vi "CoilsInit.vi"(8 "error in":errorcluster, 9 "DO Lines":tag, 10 "AO Channels":tag, 11 "Keithley USB":refnum<visa-resource-name>) -> (0 "error out":errorcluster, 1 "DO Task out":refnum<k21>, 2 "AO Task out":refnum<k21>, 3 "Keithley USB out":refnum<visa-resource-name>)   [LabVIEW 2012]
uses:
  <vilib>/DAQmx/create/channels.llb/DAQmx Create Channel (AO-Voltage-Basic).vi
  <vilib>/DAQmx/create/channels.llb/DAQmx Create Channel (DO-Digital Output).vi
  <resource>/objmgr/daqmx.rc
  Keithley KE22xx Series/Keithley KE22xx Series.lvlib
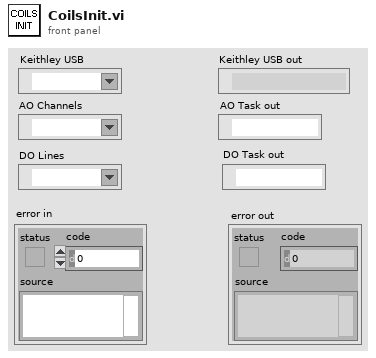
[diagram p1: front panel]
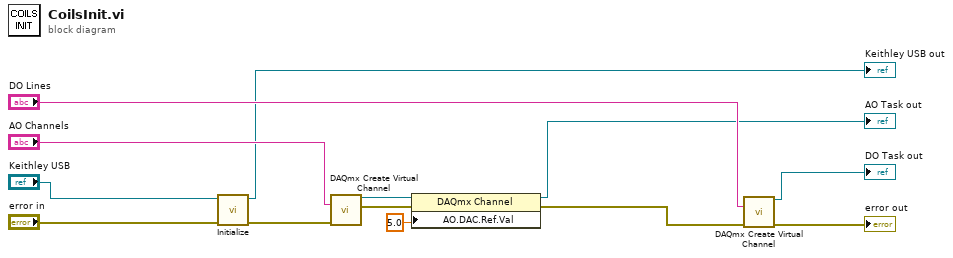
[diagram p0: block diagram]
diagram:
  n1 = call "Initialize.vi"("error in (no error)"="error in", "VISA resource name"="Keithley USB") -> ("error out"=w9:errorcluster, "VISA resource name out"=→"Keithley USB out":refnum<visa-resource-name>)  [unwired: 8 in]
  n2 = call-poly <vilib>:"DAQmx Create Virtual Channel.vi"("physical channels"="AO Channels", "error in"=w9) -> ("task out"=w12:refnum<k21>, "error out"=w11:errorcluster)  [unwired: 12 in]
  n3 = property class="DAQmx Channel"(reference=w12, error in=w11, "AO.DAC.Ref.Val"=5.0) -> (reference out=→"AO Task out":refnum<k21>, error out=w8:errorcluster)
  n4 = call-poly <vilib>:"DAQmx Create Virtual Channel.vi"("lines"="DO Lines", "error in"=w8) -> ("task out"=→"DO Task out":refnum<k21>, "error out"=→"error out":errorcluster)  [unwired: 12 in]
